vi "test Scheduled Loopback Value Overflow.vi"(8 "error in":errorcluster, 11 "TestCase in":refnum<class "Single Board 1Ch Loopback.lvclass">) -> (0 "error out":errorcluster, 3 "TestCase out":refnum<class "Single Board 1Ch Loopback.lvclass">)   [LabVIEW 2020, in "Single Board 1Ch Loopback.lvclass"]
uses:
  Single Board 1Ch Loopback.lvclass
  C:/dev/git/niveristand-custom-device-testing-tools/VeriStandTestCase/VeriStandTestCase.lvclass
  <vilib>/numeric/sub_Random U32.vi
  <vilib>/numeric/Random Number (Range) U64.vi
  <vilib>/NI VeriStand/Execution/Workspace/NI VeriStand - Set Multiple Channel Values.vi
  <vilib>/addons/_JKI Toolkits/VI Tester/TestCase.llb/TestCase.lvclass
  <vilib>/NI VeriStand/Execution/Workspace/NI_VS Workspace ExecutionAPI.lvlib
  niveristand-custom-device-testing-tools/VeriStandTestUtilities/VeriStandTestUtilities.lvlib
  C:/Program Files (x86)/National Instruments/LabVIEW 2020/vi.lib/addons/_JKI Toolkits/VI Tester/TestCase.llb/TestCase.lvclass
  C:/dev/git/niveristand-aim-arinc429-custom-device/Source/Custom Device Support/Tests/System/Single Board (CH2--CH3) Loopback/Single Board 1Ch Loopback.lvclass
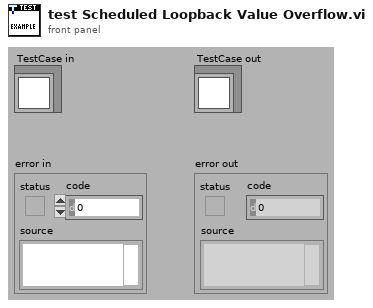
[diagram p1: front panel]
types:
  T1 = typedef "NI_VS Workspace ExecutionAPI.lvlib/WorkspaceAPI.ctl" = refnum<k24>
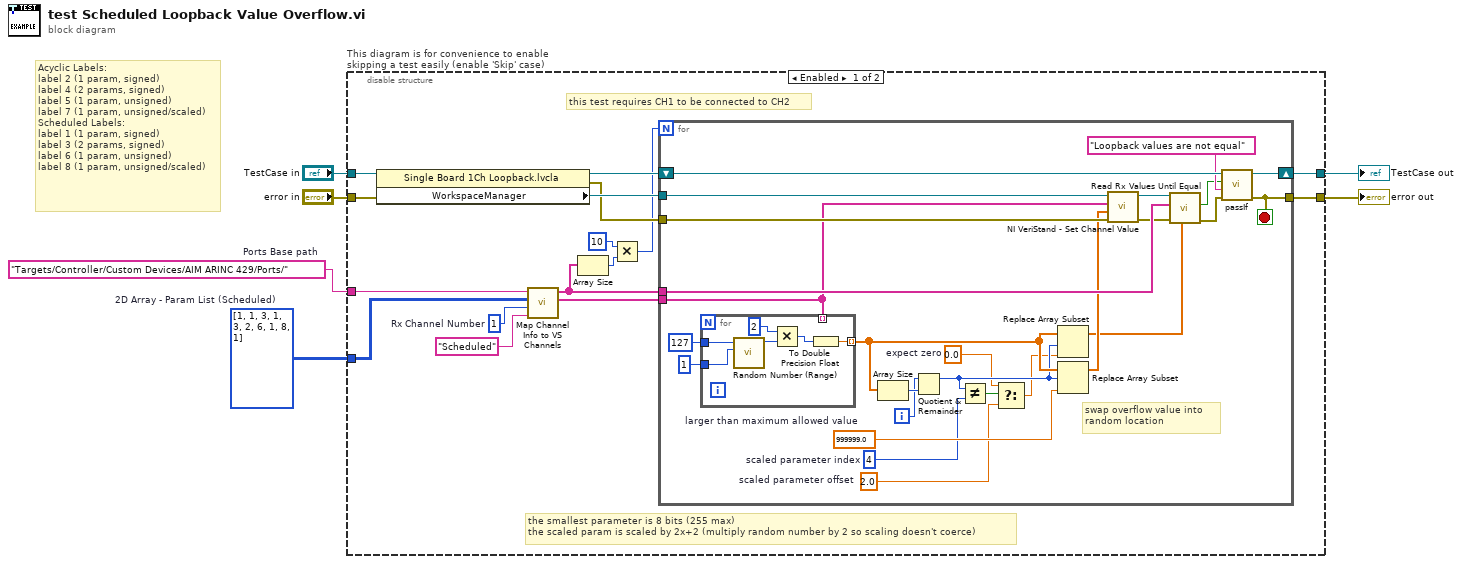
[diagram p0: block diagram]
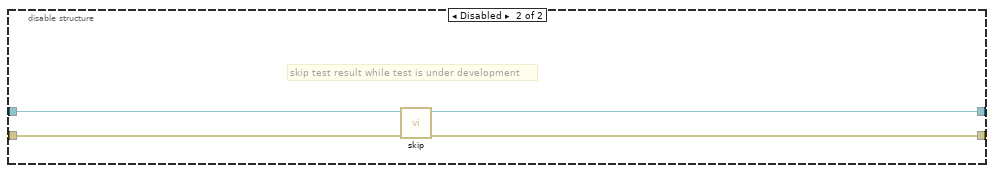
[diagram p2: hidden frame]
diagram:
  w1 = i32[][] [[1, 1], [3, 1], [3, 2], [6, 1], [8, 1]]  # 2D Array - Param List (Scheduled)
  w2 = "Targets/Controller/Custom Devices/AIM ARINC 429/Ports/"  # Ports Base path
  # "Acyclic Labels:\nlabel 2 (1 param, signed)\nlabel 4 (2 params, signed)\nlabel 5 (1 param, unsigned)\nlabel 7 (1 param, unsigned/scaled)\nScheduled Labels:\nlabel 1 (1 param, signed)\nlabel 3 (2 params, signed)\nlabel 6 (1 param, unsigned)\nlabel 8 (1 param, unsigned/scaled)"
  n1 = disable-structure "This diagram is for convenience to enable skipping a test easily (enable 'Skip' case)" shown="Enabled" {
    disable-tunnel: "TestCase in" -> [w18 w58]
    disable-tunnel: [w16 w56] -> w3
    disable-tunnel: [w15 w57] -> w5
    disable-tunnel: "error in" -> [w17 w55]
    disable-tunnel: w2 -> [w19 _]
    disable-tunnel: w1 -> [w12 _]
    frame Enabled {
      w13 = 1  # Rx Channel Number
      # "this test requires CH1 to be connected to CH2"
      # "the smallest parameter is 8 bits (255 max)\nthe scaled param is scaled by 2x+2 (multiply random number by 2 so scaling doesn't coerce)"
      n2 = property class="Single Board 1Ch Loopback.lvcla"(reference=w18, error in=w17) -> (reference out=w20:refnum<class "Single Board 1Ch Loopback.lvclass">, error out=w21:errorcluster, "WorkspaceManager"=w22:T1)
      n3 = call "Map Channel Info to VS Channels.vi"("Transfer Type"="Scheduled", "Rx Channel Number"=w13, "2D Array - Label/Param List"=w12, "VS Channel Base Port"=w19) -> ("Tx Channels Array"=w11:string[], "Rx Channels Array"=w10:string[])  [unwired: 4 in, 2 out]
      n4 = Array Size(array=w10) -> (size(s)=w9:i32)
      n5 = Multiply(x=10, y=w9) -> (x*y=w7:i32)
      n6 = for {
        N: w7 -> [_]
        tunnel: w10 -> [w41]
        tunnel: w22 -> [w35]
        tunnel: w21 -> [w40]
        tunnel: w11 -> [w34]
        shift-right: [w47] -> w16
        shift-left: w20 -> [w48]
        tunnel: [w46] -> w15
        i -> [w29]
        stop <- w46 stop-if-true
        w24 = 2.0  # scaled parameter offset
        w27 = 4  # scaled parameter index
        w25 = 0.0  # expect zero
        w42 = 999999.0  # larger than maximum allowed value
        # "swap overflow value into \nrandom location"
        n7 = for {
          tunnel: [w53] -> w30 mode=indexing
          tunnel: u64 127 ("upper bound (100)") -> [w52]
          tunnel: u64 1 ("upper bound (100)") -> [w51]
          tunnel: w34 -> [_] mode=indexing
          n8 = call-poly <vilib>:"Random Number (Range).vi"("lower bound (0)"=w51, "upper bound (100)"=w52) -> ("number"=w54:u64)  [unwired: 9 in]
          n9 = Multiply(x=u64 2, y=w54) -> (x*y=w50:u64)
          n10 = To Double Precision Float(number=w50) -> (double precision float=w53:dbl)
        }
        n11 = Array Size(array=w30) -> (size(s)=w31:i32)
        n12 = Quotient & Remainder(x=w29, y=w31) -> (x-y*floor(x/y)=w28:i32)  [unwired: 1 out]
        n13 = Not Equal?(x=w28, y=w27) -> (x != y?=w26:bool)
        n14 = Select(t=w25, s=w26, f=w24) -> (s? t:f=w23:dbl)
        n15 = Replace Array Subset(array=w30, new element=w23, index=w28) -> (w32:dbl[])
        n16 = Replace Array Subset(array=w30, new element=w42, index=w28) -> (w33:dbl[])
        n17 = call-poly <vilib>:"NI VeriStand - Set Channel Value.vi"("error in (no error)"=w40, "Values"=w33, "Channels"=w34, "WorkspaceManager in"=w35) -> ("error out"=w39:errorcluster, "WorkspaceManager out"=w36:T1)  [unwired: 6 in]
        n18 = call "Read Rx Values Until Equal.vi"("expected values"=w32, "error in"=w39, "Rx aliases"=w41, "workspace manager in"=w36) -> ("error out"=w38:errorcluster, "values equal expected"=w37:bool)  [unwired: 5 in, 1 out]
        n19 = call-dynamic "passIf.vi"("error in (no error)"=w38, "message (\"\")"="Loopback values are not equal" ("message (\"\")"), "pass"=w37, "TestCase in"=w48) -> ("error out"=w46:errorcluster, "TestCase out"=w47:refnum<class "Single Board 1Ch Loopback.lvclass">)  [unwired: 6 in]
      }
    }
    frame Disabled {
      # "skip test result while test is under development"
      n20 = call <vilib>:"skip.vi"("error in (no error)"=w55, "TestCase in"=w58) -> ("error out"=w57:errorcluster, "TestCase out"=w56:refnum<class "Single Board 1Ch Loopback.lvclass">)  [unwired: 8 in]
    }
  }
  "error out" <- w5
  "TestCase out" <- w3
